vi "Populate PWM Waveforms Entry.vi"(8 "error in":errorcluster, 9 "PWM Waveform":digitalwaveform(waveform), 10 "Channel Ident":string, 11 "DO DAQmx Fixed Freq PWM CFG in":refnum<class "DO DAQmx Fixed Freq PWM CFG.lvclass">) -> (0 "error out":errorcluster, 3 "DO DAQmx Fixed Freq PWM CFG in 2":refnum<class "DO DAQmx Fixed Freq PWM CFG.lvclass">)   [LabVIEW 2024, in "DO DAQmx Fixed Freq PWM CFG.lvclass"]
uses:
  DO DAQmx Fixed Freq PWM CFG.lvclass
  DO DAQmx Fixed Freq PWM CFG.lvclass/DO DAQmx Fixed Freq PWM CFG.ctl
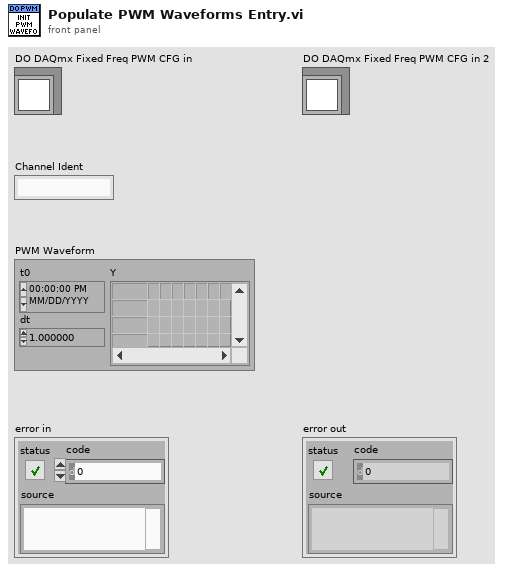
[diagram p1: front panel]
types:
  T1 = cluster{"Channel":string, "Digital Waveform":digitalwaveform}[]
  T2 = cluster{"Channel Ident":string, "PWM Waveform":digitalwaveform}
  T3 = cluster{"Channel Ident":string, "PWM Waveform":digitalwaveform}[]
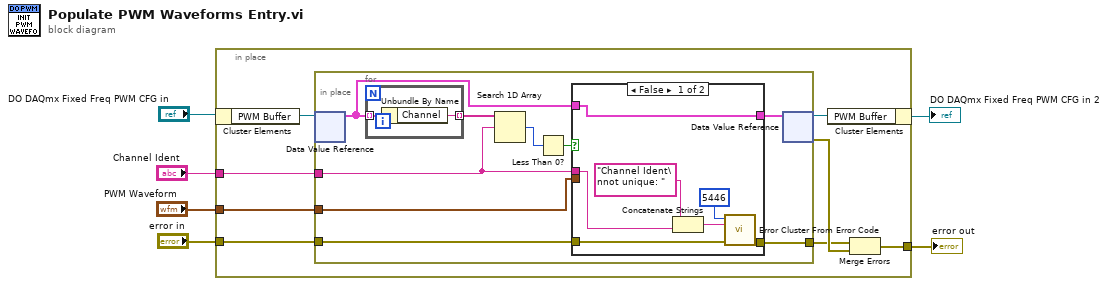
[diagram p0: block diagram]
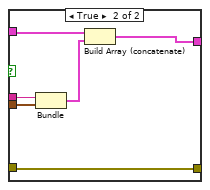
[diagram p2: hidden frame]
diagram:
  n1 = in-place {
    in-place-border: "Channel Ident" -> [w14]
    in-place-border: "error in" -> [w8]
    in-place-border: "PWM Waveform" -> [w13]
    in-place-border: [w12] -> w3
    n2 = in-place-cluster #1("DO DAQmx Fixed Freq PWM CFG in") -> ("PWM Buffer"=w10:refnum<data-value>)
    n3 = in-place {
      in-place-border: w14 -> [w19]
      in-place-border: w13 -> [w18]
      in-place-border: w8 -> [w16]
      in-place-border: [w15] -> w7
      n4 = in-place-dvr #2(w10) -> (w20:T1)  [unwired: 1 out]
      n5 = for {
        tunnel: w20 -> [w38] mode=indexing
        tunnel: [w37] -> w23 mode=indexing
        n6 = Unbundle By Name(w38) -> ("Channel"=w37:string)
      }
      n7 = Search 1D Array(1D array=w23, element=w19) -> (index of element=w22:i32)  [unwired: 1 in]
      n8 = Less Than 0?(x=w22) -> (x < 0?=w21:bool)
      n9 = case shown="False" w21 {
        tunnel: w20 -> [w24 w34]
        tunnel: w19 -> [w26 w36]
        tunnel: w18 -> [_ w35]
        tunnel: [w24 w32] -> w17
        tunnel: w16 -> [w30 w31]
        tunnel: [w25 w31] -> w15
        frame False {
          n10 = Concatenate Strings("Channel Ident\nnot unique: ", w26) -> (w28:string)
          n11 = call <vilib>:"Error Cluster From Error Code.vi"("error in (no error)"=w30, "error message (\"\")"=w28, "error code (0)"=5446) -> ("error out"=w25:errorcluster)  [unwired: 6 in]
        }
        frame True {
          n12 = Bundle("Channel Ident"=w36, "PWM Waveform"=w35) -> (w33:T2)  [unwired: 1 in]
          n13 = Build Array (concatenate)(w34, w33) -> (w32:T3)
        }
      }
      n14 = in-place-dvr #2(w17) -> (w9:refnum<data-value>, w11:errorcluster)
    }
    n15 = in-place-cluster #1("PWM Buffer"=w9) -> (→"DO DAQmx Fixed Freq PWM CFG in 2":refnum<class "DO DAQmx Fixed Freq PWM CFG.lvclass">)
    n16 = Merge Errors(w7, w11) -> (w12:errorcluster)
  }
  "error out" <- w3
